vi "run.vi"   [LabVIEW 2017, in "rethinkdb.lvlib"]
uses:
  rethinkdb.lvlib
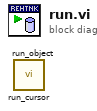
[diagram p0: block diagram]
diagram:
  n1 = call "run_cursor.vi"() -> ()  [unwired: 9 in, 3 out]
  n2 = call "run_object.vi"() -> ()  [unwired: 9 in, 3 out]
